vi "CD.vi"(1 "dec dig":T2) -> (0 "Bin":T1)   [LabVIEW 2012]
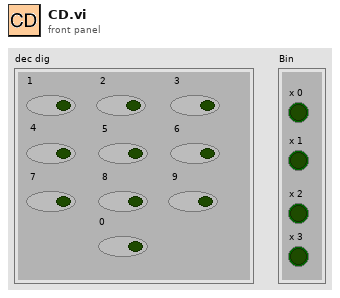
[diagram p1: front panel]
types:
  T1 = cluster{"x 0":bool, "x 1":bool, "x 2":bool, "x 3":bool}
  T2 = cluster{"0":bool, "1":bool, " 2":bool, " 3":bool, " 4":bool, " 5":bool, " 6":bool, " 7":bool, " 8":bool, " 9":bool}
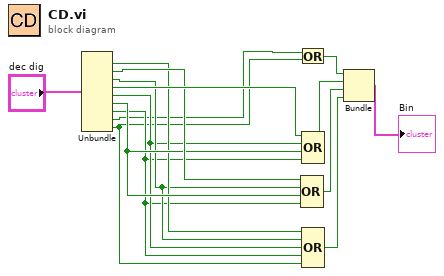
[diagram p0: block diagram]
diagram:
  n1 = Unbundle("dec dig") -> ("1"=w7:bool, "2"=w9:bool, "3"=w6:bool, "4"=w10:bool, "5"=w5:bool, "6"=w8:bool, "7"=w4:bool, "8"=w2:bool, "9"=w1:bool)  [unwired: 1 out]
  n2 = Or(x=w2, y=w1) -> (x .or. y?=w3:bool)
  n3 = Compound Arithmetic op=OR(w9, w6, w8, w4) -> (w12:bool)
  n4 = Compound Arithmetic op=OR(w10, w5, w8, w4) -> (w11:bool)
  n5 = Compound Arithmetic op=OR(w7, w6, w5, w4, w1) -> (w13:bool)
  n6 = Bundle(w3, w11, w12, w13) -> (→"Bin":cluster{bool, bool, bool, bool})  [unwired: 1 in]
